vi "ssh_fgv.vi"(0 "?":T2, 1 "User Name":string="git", 2 "Input":string, 3 "Host Address":string="10.13.7.56", 4 "Password":string="1234", 5 "error in":errorcluster) -> (7 "output_new":string, 8 "error out":errorcluster)   [LabVIEW 2016, in "labssh_thijs.lvlib"]
uses:
  labssh_thijs.lvlib
  state machine.ctl
  LabSSH/LabSSH/LabSSH/bin/Debug/State Date..cluster.ctl
  C:/Users/thosman/Documents/Development/Labview/ssh in labview/LabSSH/LabSSH/LabSSH/bin/Debug/LabSSH.dll
  LabSSH/LabSSH/LabSSH/bin/Debug/LabSSH.dll
  C:/Users/thosman/Documents/Development/Labview/ssh in labview/LabSSH/LabSSH/References/Renci.SshNet.dll
  LabSSH/LabSSH/References/Renci.SshNet.dll
  LabSSH LabVIEW/LabSSH.lvlib
panel:
  in  "?":T1
  out "state":T2
  out "stop":bool
  out "Output":string
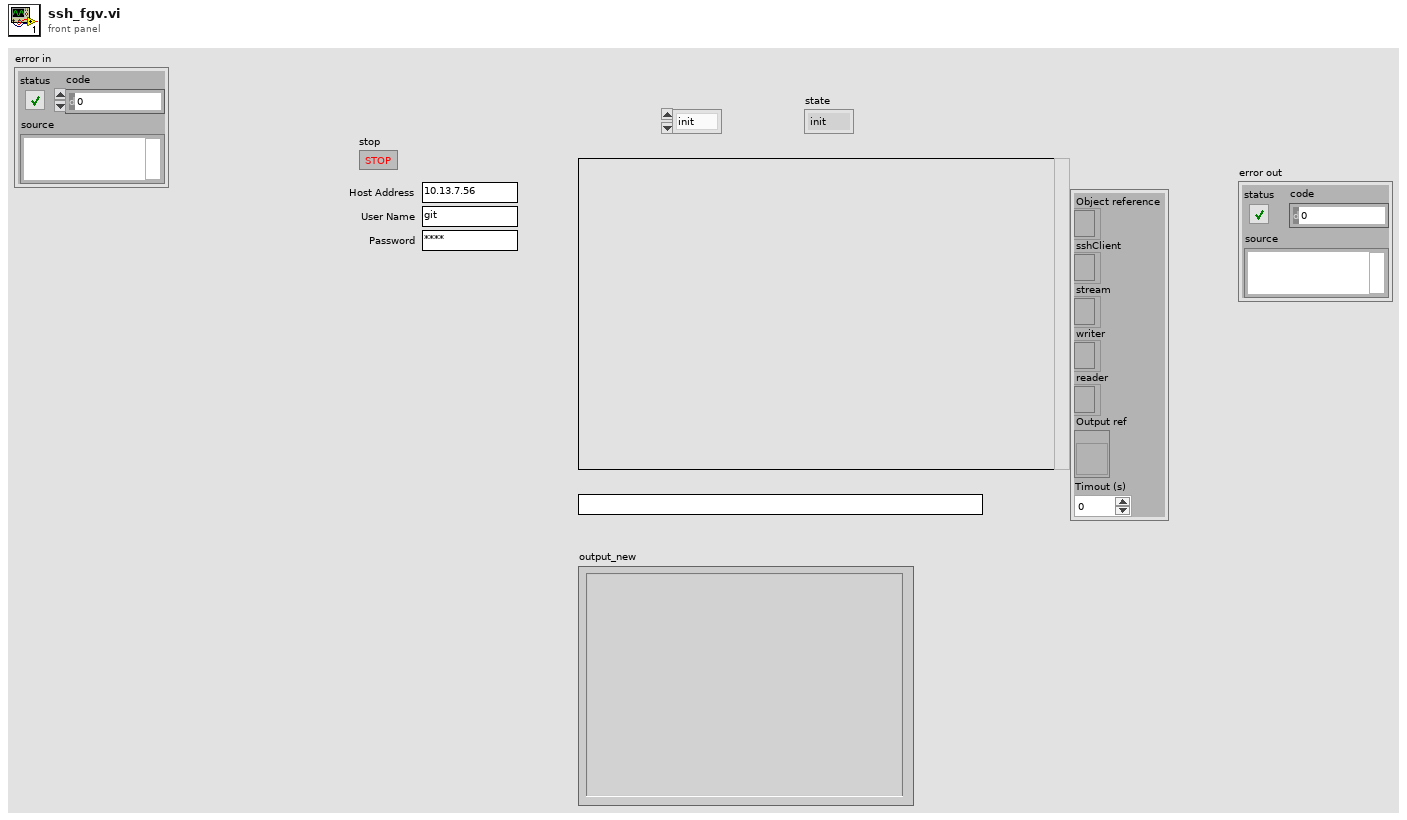
[diagram p1: front panel]
types:
  T1 = typedef "labssh_thijs.lvlib/LabSSH.lvlib/State Date..cluster.ctl" = cluster{"Object reference":refnum<k24>, "sshClient":refnum<k24>, "stream":refnum<k24>, "writer":refnum<k24>, "reader":refnum<k24>, "Output ref":refnum<vi>, "Timout (s)":i32}
  T2 = typedef "labssh_thijs.lvlib/state machine.ctl" = enum16{"init", "connect", "execute", "close", "exit", "read"}
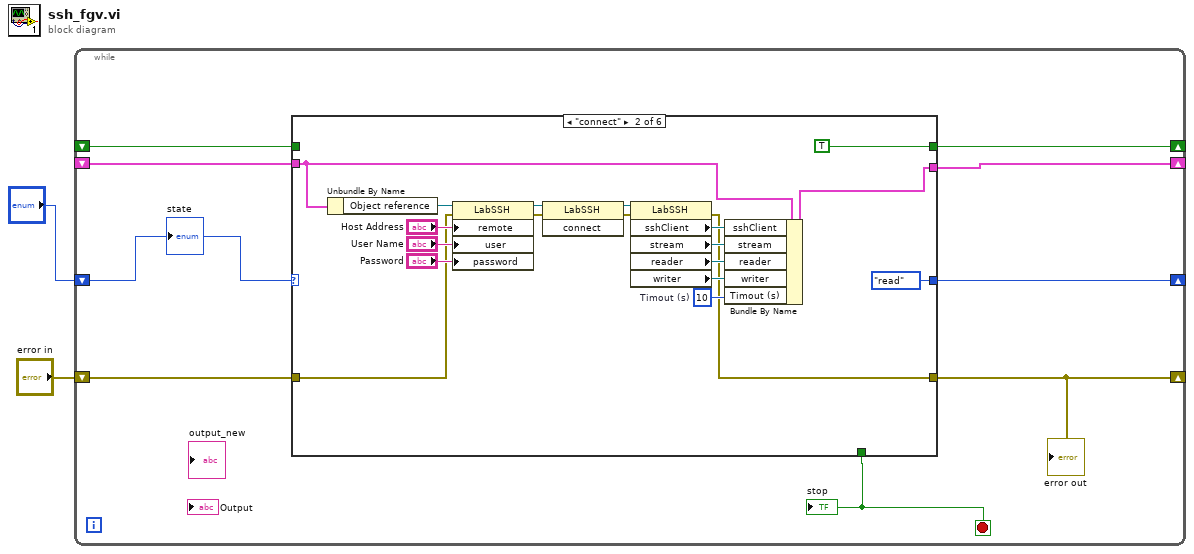
[diagram p0: block diagram]
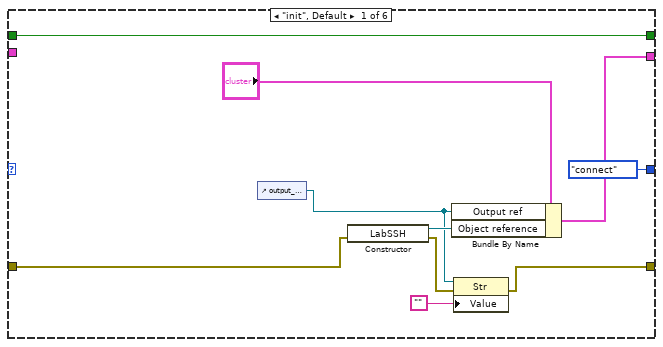
[diagram p2: hidden frame]
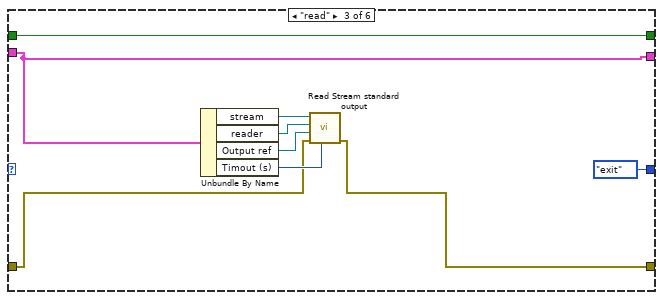
[diagram p3: hidden frame]
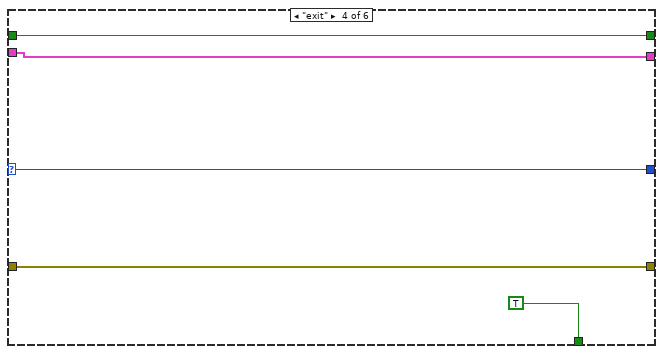
[diagram p4: hidden frame]
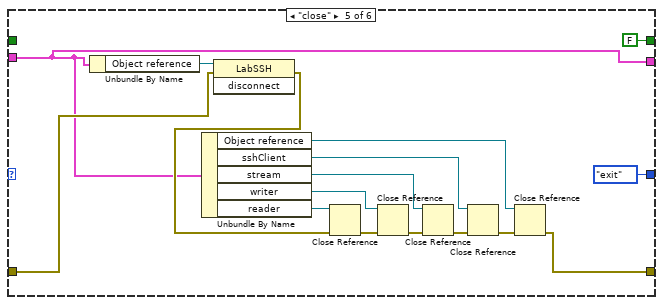
[diagram p5: hidden frame]
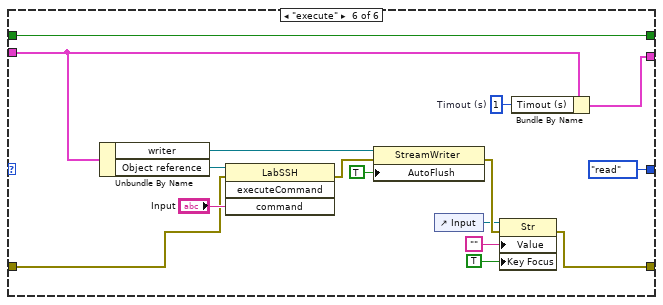
[diagram p6: hidden frame]
diagram:
  n1 = while {
    shift-right: [w9] -> _
    shift-left: "error in" -> [w10]
    shift-right: [w8] -> _
    shift-left: _ -> [w3]
    shift-right: [w6] -> _
    shift-left: "?" -> [w11]
    shift-right: [w5] -> _
    shift-left: _ -> [w4]
    stop <- w7 stop-if-true
    n2 = case shown="\"connect\"" w11 {
      selector: w11 -> [_ _ _ w52 _ _]
      tunnel: w3 -> [_ w27 w42 w51 w55 w73]
      tunnel: w10 -> [w17 w25 w45 w53 w57 w72]
      tunnel: [w16 w24 w41 w53 w56 w71] -> w9
      tunnel: [w15 w26 w42 w51 w55 w75] -> w8
      tunnel: [_ _ _ TRUE ("stop") _ _] -> w7
      tunnel: [state_machine."connect" state_machine."read" state_machine."exit" w52 state_machine."exit" state_machine."read"] -> w6
      tunnel: [w14 TRUE ("stop") w43 w50 FALSE ("stop") w74] -> w5
      tunnel: w4 -> [w14 _ w43 w50 _ w74]
      frame "init", Default {
        n3 = control-ref of="output_new"() -> (w18:refnum<vi>)
        n4 = constructor class="LabSSH"(error in=w17) -> (reference out=w19:refnum<k24>, error out=w20:errorcluster)  [unwired: 2 in, 1 out]
        n5 = Bundle By Name(cluster="?", "Output ref"=w18, "Object reference"=w19) -> (w15:T1)
        n6 = property class="Str"(reference=w18, error in=w20, "Value"="") -> (error out=w16:errorcluster)  [unwired: 1 out]
      }
      frame "connect" {
        w40 = 10  # Timout (s)
        n7 = Unbundle By Name(w27) -> ("Object reference"=w28:refnum<k24>)
        n8 = property class="LabSSH"(reference=w28, error in=w25, "remote"="Host Address", "user"="User Name", "password"="Password") -> (reference out=w35:refnum<k24>, error out=w36:errorcluster)
        n9 = invoke class="LabSSH" method="connect"(reference=w35, error in=w36) -> (reference out=w29:refnum<k24>, error out=w30:errorcluster)  [unwired: 1 in, 1 out]
        n10 = property class="LabSSH"(reference=w29, error in=w30) -> (error out=w24:errorcluster, "sshClient"=w31:refnum<k24>, "stream"=w32:refnum<k24>, "reader"=w33:refnum<k24>, "writer"=w34:refnum<k24>)  [unwired: 1 out]
        n11 = Bundle By Name(cluster=w27, "sshClient"=w31, "stream"=w32, "reader"=w33, "writer"=w34, "Timout (s)"=w40) -> (w26:T1)
      }
      frame "read" {
        n12 = Unbundle By Name(w42) -> ("stream"=w46:refnum<k24>, "reader"=w47:refnum<k24>, "Output ref"=w49:refnum<vi>, "Timout (s)"=w48:i32)
        n13 = call "Read Stream standard output.vi"("Timout (s)"=w48, "error in (no error)"=w45, "Output ref"=w49, "reader"=w47, "stream"=w46) -> ("error out"=w41:errorcluster)  [unwired: 6 in]
      }
      frame "exit" {
      }
      frame "close" {
        n14 = Unbundle By Name(w55) -> ("Object reference"=w60:refnum<k24>)
        n15 = Unbundle By Name(w55) -> ("Object reference"=w69:refnum<k24>, "sshClient"=w68:refnum<k24>, "stream"=w67:refnum<k24>, "writer"=w66:refnum<k24>, "reader"=w65:refnum<k24>)
        n16 = invoke class="LabSSH" method="disconnect"(reference=w60, error in=w57) -> (error out=w58:errorcluster)  [unwired: 1 in, 2 out]
        n17 = Close Reference(reference=w65, error in (no error)=w58) -> (error out=w64:errorcluster)
        n18 = Close Reference(reference=w66, error in (no error)=w64) -> (error out=w61:errorcluster)
        n19 = Close Reference(reference=w67, error in (no error)=w61) -> (error out=w63:errorcluster)
        n20 = Close Reference(reference=w68, error in (no error)=w63) -> (error out=w62:errorcluster)
        n21 = Close Reference(reference=w69, error in (no error)=w62) -> (error out=w56:errorcluster)
      }
      frame "execute" {
        w82 = 1  # Timout (s)
        n22 = Unbundle By Name(w73) -> ("writer"=w79:refnum<k24>, "Object reference"=w77:refnum<k24>)
        n23 = invoke class="LabSSH" method="executeCommand"(reference=w77, error in=w72, "command"="Input") -> (error out=w81:errorcluster)  [unwired: 1 in, 3 out]
        n24 = property class="StreamWriter"(reference=w79, error in=w81, "AutoFlush"=TRUE) -> (error out=w84:errorcluster)  [unwired: 1 out]
        n25 = control-ref of="Input"() -> (w83:refnum<vi>)
        n26 = property class="Str"(reference=w83, error in=w84, "Value"="", "Key Focus"=TRUE) -> (error out=w71:errorcluster)  [unwired: 1 out]
        n27 = Bundle By Name(cluster=w73, "Timout (s)"=w82) -> (w75:T1)
      }
    }
    "stop" <- w7
    "error out" <- w9
    "state" <- w11
  }
